vi "Unpack Analog Command.vi"(8 "error in (no error)":errorcluster, 9 "Data":variant, 10 "Type":string, 11 "Module in":refnum<class "Module.lvclass">) -> (0 "error out":errorcluster, 1 "Remote":bool, 2 "CmdAnalogMultiple":T2, 3 "Module out":refnum<class "Module.lvclass">, 5 "TcpPayload":T1)   [LabVIEW 2023, in "Volatus.lvlib" / "Module.lvclass"]
uses:
  Module.lvclass
  Module.lvclass/Module.ctl
  messages/CmdAnalogMultiple/Class/Msg.lvclass
  messages/CmdAnalog/Data.ctl
  messages/CmdAnalog/CmdAnalog.lvlib
  messages/CmdAnalogMultiple/Data.ctl
  messages/CmdAnalogMultiple/CmdAnalogMultiple.lvlib
  C:/dev/volatus/mts-volatus-super/libs/lv-volatus/messages/CmdAnalogMultiple/Class/Msg.lvclass
  C:/dev/volatus/mts-volatus-super/libs/lv-protoc/LV-Proto/Message/Message.lvclass
  lv-vecto/Vecto/proto/TcpPayload/Data.ctl
  lv-vecto/Vecto/proto/TcpPayload/TcpPayload.lvlib
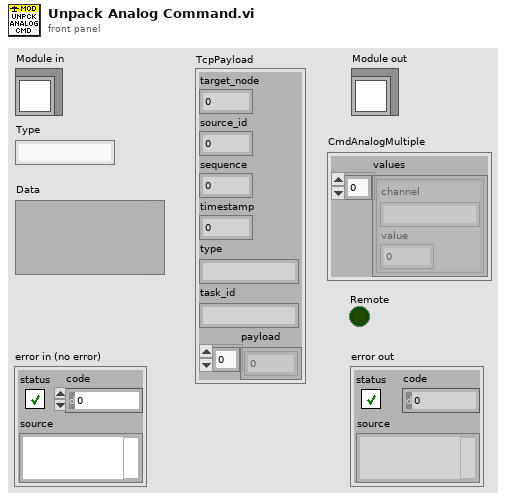
[diagram p1: front panel]
types:
  T1 = typedef "TcpPayload.lvlib/Data.ctl" = cluster{"target_node":u32, "source_id":u32, "sequence":u32, "timestamp":i64, "type":string, "task_id":string, "payload":u8[]}
  T2 = typedef "CmdAnalogMultiple.lvlib/Data.ctl" = cluster{"values":T3[]}
  T3 = typedef "CmdAnalog.lvlib/Data.ctl" = cluster{"channel":string, "value":dbl}
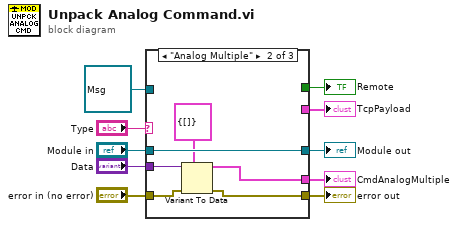
[diagram p0: block diagram]
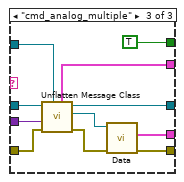
[diagram p3: hidden frame]
diagram:
  n1 = case shown="\"Analog Multiple\"" "Type" {
    tunnel: "Data" -> [_ w17 w26]
    tunnel: "error in (no error)" -> [w11 w16 w25]
    tunnel: "Module in" -> [w12 w18 w29]
    tunnel: [w12 w18 w28] -> w6
    tunnel: [_ _ TRUE] -> w5
    tunnel: [w11 w15 w20] -> w4
    tunnel: refnum<class "Msg.lvclass"> refnum ("CmdAnalogMultiple.lvlib:Msg.lvclass") -> [_ _ w24]
    tunnel: [_ _ w23] -> w2
    tunnel: [_ w13 w19] -> w1
    frame Default {
    }
    frame "Analog Multiple" {
      n2 = Variant To Data(error in=w16, type=T2 {"values"=[]} ("Data"), Variant=w17) -> (data=w13:T2, error out=w15:errorcluster)
    }
    frame "cmd_analog_multiple" {
      n3 = call "Unflatten Message Class.vi"("Message Type"=w24, "error in (no error)"=w25, "Data"=w26, "Module in"=w29) -> ("error out"=w21:errorcluster, "Message"=w22:refnum<class "Msg.lvclass">, "Module out"=w28:refnum<class "Module.lvclass">, "TcpPayload"=w23:T1)  [unwired: 4 in]
      n4 = call "Data.vi"("error in (no error)"=w21, "PB Msg Template in"=w22) -> ("error out"=w20:errorcluster, "Data"=w19:T2)  [unwired: 7 in, 1 out]
    }
  }
  "error out" <- w4
  "Module out" <- w6
  "CmdAnalogMultiple" <- w1
  "Remote" <- w5
  "TcpPayload" <- w2
